vi "Add Channel Reference.vi"(8 "error in (no error)":errorcluster, 10 "Channel Path":string, 11 "RT Sequence Ref in":refnum<k24>) -> (0 "error out":errorcluster, 3 "RT Sequence Ref out":refnum<k24>)   [LabVIEW 2016, in "RT Sequence Creator API.lvlib"]
uses:
  RT Sequence Creator API.lvlib
  NationalInstruments.VeriStand.RealTimeSequenceDefinitionApi
  NationalInstruments.VeriStand.DataTypes
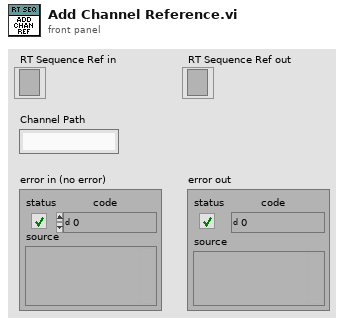
[diagram p1: front panel]
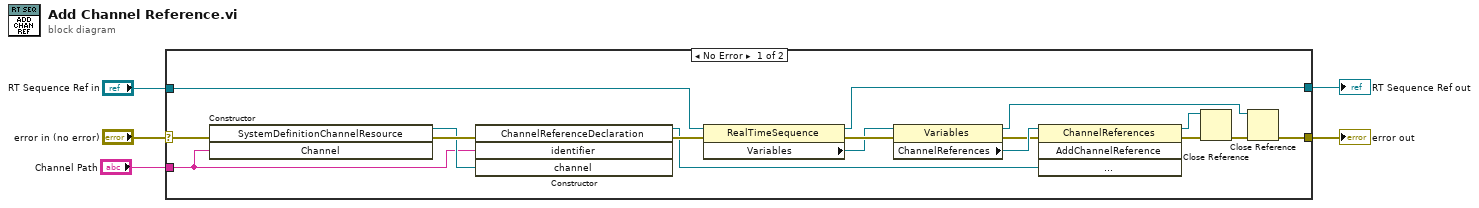
[diagram p0: block diagram]
diagram:
  n1 = case shown="No Error" "error in (no error)" {
    selector: "error in (no error)" -> [w7 w23]
    tunnel: "RT Sequence Ref in" -> [w21 w24]
    tunnel: [w14 w23] -> w3
    tunnel: [w20 w24] -> w2
    tunnel: "Channel Path" -> [w6 _]
    frame No Error {
      n2 = constructor class="SystemDefinitionChannelResource"(error in=w7, "Channel"=w6) -> (reference out=w9:refnum<k24>, error out=w10:errorcluster)  [unwired: 2 in, 2 out]
      n3 = constructor class="ChannelReferenceDeclaration"(error in=w10, "identifier"=w6, "channel"=w9) -> (reference out=w8:refnum<k24>, error out=w11:errorcluster)  [unwired: 2 in, 3 out]
      n4 = property class="RealTimeSequence"(reference=w21, error in=w11) -> (reference out=w20:refnum<k24>, error out=w22:errorcluster, "Variables"=w19:refnum<k24>)
      n5 = property class="Variables"(reference=w19, error in=w22) -> (reference out=w12:refnum<k24>, error out=w17:errorcluster, "ChannelReferences"=w18:refnum<k24>)
      n6 = invoke class="ChannelReferences" method="AddChannelReference"(reference=w18, error in=w17, "channelRef"=w8) -> (reference out=w13:refnum<k24>, error out=w16:errorcluster)  [unwired: 1 in, 2 out]
      n7 = Close Reference(reference=w13, error in (no error)=w16) -> (error out=w15:errorcluster)
      n8 = Close Reference(reference=w12, error in (no error)=w15) -> (error out=w14:errorcluster)
    }
    frame Error {
    }
  }
  "RT Sequence Ref out" <- w2
  "error out" <- w3
